vi "SUB ZeroPhaseFilter.vi"(10 "Options":T2={"Name"=0, "f-"=1.0, "f+"=1000.0, "order"=1.0, "filter type"=enum."Bandpass"} {"Name" items=["Butterworth", "Elliptic", "Chebyshev", "Bessel"]}, 11 "Prefilter":waveform(dbl)) -> (3 "FilteredWaveform":waveform(dbl))   [LabVIEW 2017]
uses:
  <vilib>/Analysis/3filter.llb/Filter Passband Type.ctl
  <vilib>/Analysis/3filter.llb/Butterworth Filter (DBL).vi
  <vilib>/Analysis/3filter.llb/Chebyshev Filter (DBL).vi
  <vilib>/Analysis/3filter.llb/Bessel Filter (DBL).vi
  <vilib>/Analysis/3filter.llb/Elliptic Filter (DBL).vi
  <vilib>/Analysis/NI_AALBase.lvlib
panel:
  out "Numeric":i32
  out "Ring Text.Text":string
  in  "filter type":T1=enum."Bandpass"
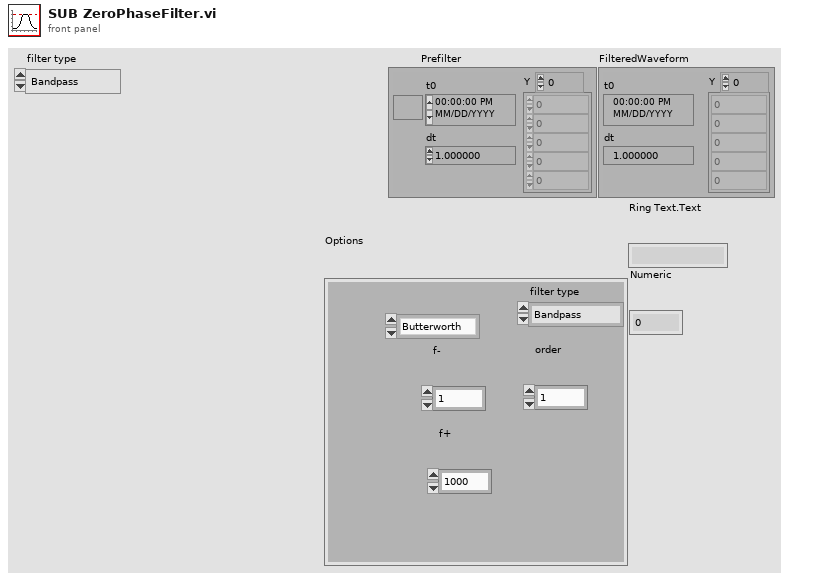
[diagram p1: front panel]
types:
  T1 = typedef "NI_AALBase.lvlib/Filter Passband Type.ctl" = enum32{"Lowpass", "Highpass", "Bandpass", "Bandstop"}
  T2 = cluster{"Name":u16, "f-":dbl, "f+":dbl, "order":dbl, "filter type":T1}
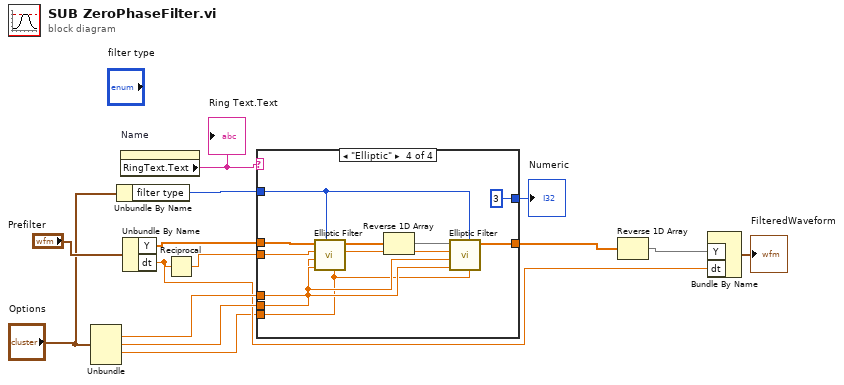
[diagram p0: block diagram]
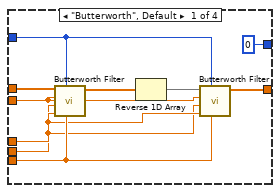
[diagram p2: hidden frame]
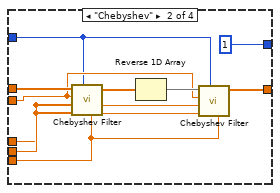
[diagram p3: hidden frame]
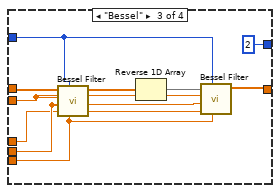
[diagram p4: hidden frame]
diagram:
  n1 = Unbundle("Options") -> ("f-"=w7:dbl, "f+"=w6:dbl, "order"=w2:dbl)  [unwired: 2 out]
  n2 = Unbundle By Name("Options") -> ("filter type"=w4:T1)
  n3 = property on="Name" class="Ring (strict)"() -> ("RingText.Text"=w8:string)  [unwired: 2 in, 2 out]
  "Ring Text.Text" <- w8
  n4 = Unbundle By Name("Prefilter") -> ("Y"=w14:dbl[], "dt"=w3:dbl)
  n5 = Reciprocal(x=w3) -> (1/x=w10:dbl)
  n6 = case shown="\"Elliptic\"" w8 {
    tunnel: w14 -> [w24 w34 w44 w51]
    tunnel: [w22 w33 w41 w52] -> w13
    tunnel: w10 -> [w21 w30 w40 w50]
    tunnel: w7 -> [w18 w28 w38 w49]
    tunnel: w6 -> [w17 w29 w39 w48]
    tunnel: w2 -> [w19 w27 w37 w47]
    tunnel: w4 -> [w16 w26 w36 w46]
    tunnel: [0 1 2 3] -> w1
    frame "Butterworth", Default {
      n7 = call-poly <vilib>:"Butterworth Filter.vi"("order"=w19, "filter type"=w16, "low cutoff freq: fl"=w18, "high cutoff freq: fh"=w17, "sampling freq: fs"=w21, "X"=w24) -> ("Filtered X"=w20:dbl[])  [unwired: 2 in, 1 out]
      n8 = Reverse 1D Array(array=w20) -> (reversed array=w23:dbl[])
      n9 = call-poly <vilib>:"Butterworth Filter.vi"("order"=w19, "filter type"=w16, "low cutoff freq: fl"=w18, "high cutoff freq: fh"=w17, "sampling freq: fs"=w21, "X"=w23) -> ("Filtered X"=w22:dbl[])  [unwired: 2 in, 1 out]
    }
    frame "Chebyshev" {
      n10 = call-poly <vilib>:"Chebyshev Filter.vi"("order"=w27, "filter type"=w26, "low cutoff freq: fl"=w28, "high cutoff freq: fh"=w29, "sampling freq: fs"=w30, "X"=w34) -> ("Filtered X"=w31:dbl[])  [unwired: 4 in, 1 out]
      n11 = Reverse 1D Array(array=w31) -> (reversed array=w32:dbl[])
      n12 = call-poly <vilib>:"Chebyshev Filter.vi"("order"=w27, "filter type"=w26, "low cutoff freq: fl"=w28, "high cutoff freq: fh"=w29, "sampling freq: fs"=w30, "X"=w32) -> ("Filtered X"=w33:dbl[])  [unwired: 4 in, 1 out]
    }
    frame "Bessel" {
      n13 = call-poly <vilib>:"Bessel Filter.vi"("order"=w37, "filter type"=w36, "low cutoff freq: fl"=w38, "high cutoff freq: fh"=w39, "sampling freq: fs"=w40, "X"=w44) -> ("Filtered X"=w43:dbl[])  [unwired: 2 in, 1 out]
      n14 = Reverse 1D Array(array=w43) -> (reversed array=w42:dbl[])
      n15 = call-poly <vilib>:"Bessel Filter.vi"("order"=w37, "filter type"=w36, "low cutoff freq: fl"=w38, "high cutoff freq: fh"=w39, "sampling freq: fs"=w40, "X"=w42) -> ("Filtered X"=w41:dbl[])  [unwired: 2 in, 1 out]
    }
    frame "Elliptic" {
      n16 = call-poly <vilib>:"Elliptic Filter.vi"("order"=w47, "passband ripple (dB)"=w46, "low cutoff freq: fl"=w49, "high cutoff freq: fh"=w48, "sampling freq: fs"=w50, "X"=w51) -> ("Filtered X"=w54:dbl[])  [unwired: 4 in, 1 out]
      n17 = Reverse 1D Array(array=w54) -> (reversed array=w53:dbl[])
      n18 = call-poly <vilib>:"Elliptic Filter.vi"("order"=w47, "filter type"=w46, "low cutoff freq: fl"=w49, "high cutoff freq: fh"=w48, "sampling freq: fs"=w50, "X"=w53) -> ("Filtered X"=w52:dbl[])  [unwired: 4 in, 1 out]
    }
  }
  "Numeric" <- w1
  n19 = Reverse 1D Array(array=w13) -> (reversed array=w12:dbl[])
  n20 = Bundle By Name("Y"=w12, "dt"=w3) -> (→"FilteredWaveform":waveform(dbl))  [unwired: 1 in]
